vi "RemoveDust.vi"(8 "error in (no error)":errorcluster, 10 "Dust removal data":T1={"Dilate data"={"Operation"=enum."Erode", "Structuring Element"=[[1, 1, 1], [1, 1, 1], [1, 1, 1]], "Number of iterations (1)"=1, "Square/Hexa (Square)"=TRUE}, "Threshold data"={"Method (clustering)"=0, "Look For (Bright Objects)"=1, "Range"={"Lower value"=128.0, "Upper value"=255.0}, "Replace Value"=1.0}} {"Threshold data"."Look For (Bright Objects)" items=["Bright Objects", "Dark Objects"]; "Threshold data"."Method (clustering)" items=["clustering", "entropy", "metric", "moments", "inter-class variance"]}, 11 "Image in":T2(plugin-control)) -> (0 "error out":errorcluster, 3 "Image out":T2(plugin-control))   [LabVIEW 2019]
uses:
  <vilib>/vision/NI_Vision_Development_Module.lvlib
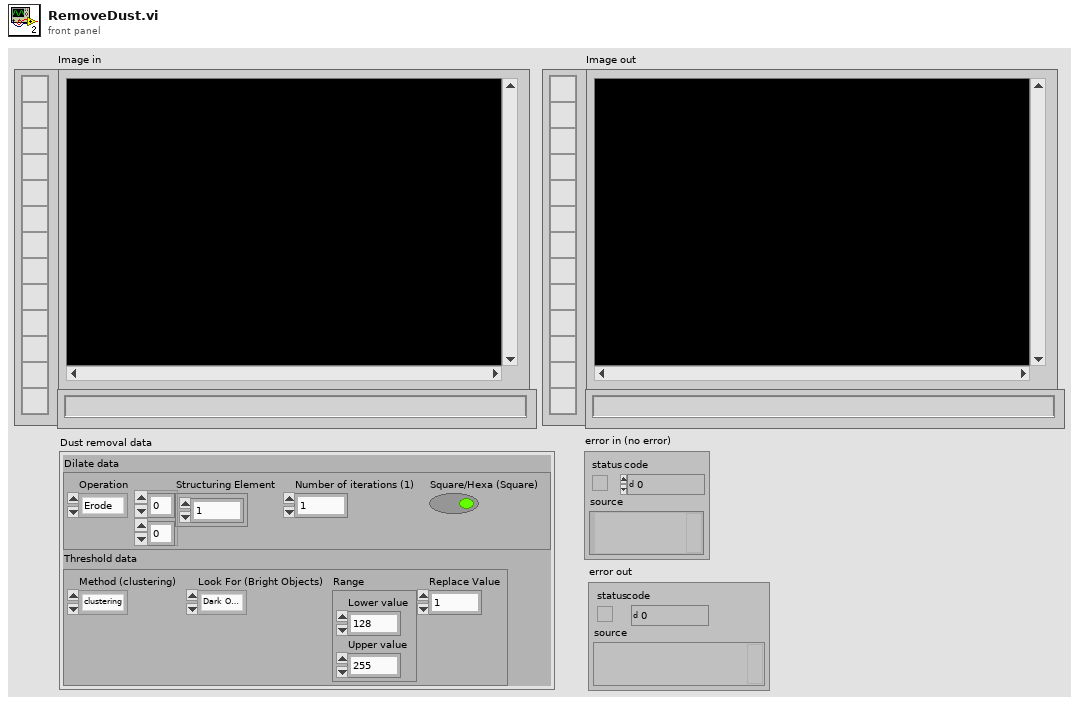
[diagram p1: front panel]
types:
  T1 = cluster{"Dilate data":cluster{"Operation":enum32{"AutoM", "Close", "Dilate", "Erode", "Gradient", "Gradient out", "Gradient in", "Hit miss", "Open", "PClose", "POpen", "Thick", "Thin"}, "Structuring Element":i32[][], "Number of iterations (1)":i32, "Square/Hexa (Square)":bool}, "Threshold data":cluster{"Method (clustering)":i32, "Look For (Bright Objects)":u32, "Range":cluster{"Lower value":sgl, "Upper value":sgl}, "Replace Value":sgl}}
  T2 = typedef "IMAQ Image.ctl" = refnum<image>
  T3 = enum32{"AutoM", "Close", "Dilate", "Erode", "Gradient", "Gradient out", "Gradient in", "Hit miss", "Open", "PClose", "POpen", "Thick", "Thin"}
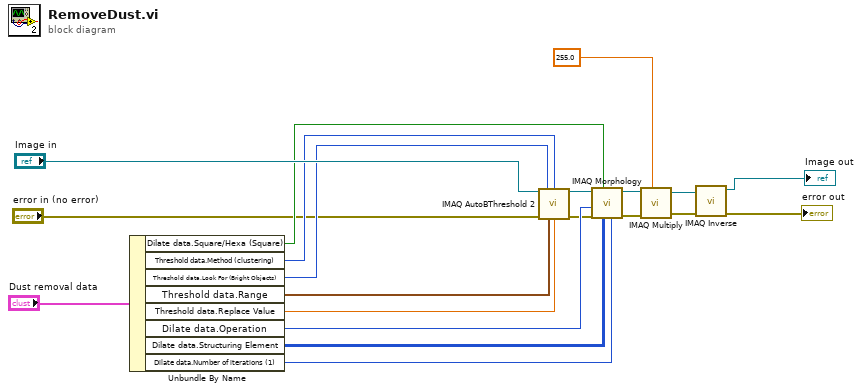
[diagram p0: block diagram]
diagram:
  n1 = Unbundle By Name("Dust removal data") -> ("Dilate data.Square/Hexa (Square)"=w6:bool, "Threshold data.Method (clustering)"=w5:i32, "Threshold data.Look For (Bright Objects)"=w4:u32, "Threshold data.Range"=w7:cluster{"Lower value":sgl, "Upper value":sgl}, "Threshold data.Replace Value"=w16:sgl, "Dilate data.Operation"=w20:T3, "Dilate data.Structuring Element"=w19:i32[][], "Dilate data.Number of iterations (1)"=w18:i32)
  n2 = call "IMAQ AutoBThreshold 2"("Image Src"="Image in", "Look For (Bright Objects)"=w4, "Method (clustering)"=w5, "error in (no error)"="error in (no error)", "Threshold Limits"=w7, "Replace Value (1)"=w16) -> ("Image Dst Out"=w3:T2, "error out"=w17:errorcluster)  [unwired: 7 in, 1 out]
  n3 = call "IMAQ Morphology"("Number of iterations (1)"=w18, "Structuring Element"=w19, "Square/Hexa (Square)"=w6, "error in (no error)"=w17, "Operation"=w20, "Image Src"=w3) -> ("error out"=w14:errorcluster, "Image Dst Out"=w13:T2)  [unwired: 4 in]
  n4 = call "IMAQ Multiply"("Image Src A"=w13, "Constant"=255.0, "error in (no error)"=w14) -> ("Image Dst Out"=w9:T2, "error out"=w11:errorcluster)  [unwired: 4 in]
  n5 = call "IMAQ Inverse"("error in (no error)"=w11, "Image Src"=w9) -> ("error out"=→"error out":errorcluster, "Image Dst Out"=→"Image out":T2)  [unwired: 8 in]
